vi "CohortRegister.vi"(10 "Action":enum16{"Set", "Get", "Del"}(ring), 11 "Cohort Index":u8) -> (3 "New Index":u8)   [LabVIEW 2012, in "StimulCtrls.lvlib"]
uses:
  StimulCtrls.lvlib
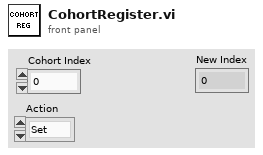
[diagram p1: front panel]
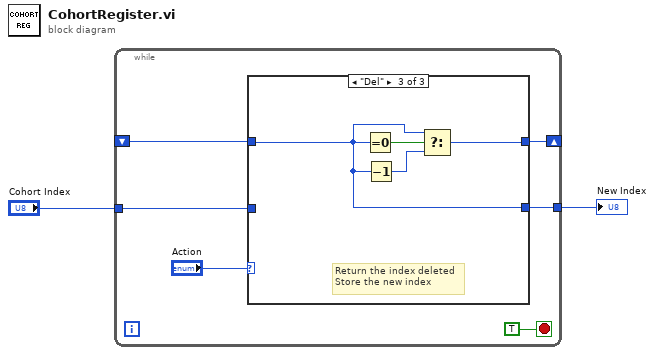
[diagram p0: block diagram]
diagram:
  n1 = while {
    tunnel: "Cohort Index" -> [w4]
    shift-right: [w7] -> _
    shift-left: _ -> [w6]
    tunnel: [w3] -> w1
    stop <- TRUE stop-if-true
    n2 = case shown="\"Del\"" "Action" {
      tunnel: [w9 w10 w12] -> w7
      tunnel: w4 -> [w9 _ _]
      tunnel: w6 -> [_ w10 w11]
      tunnel: [w9 w10 w11] -> w3
      frame "Set", Default {
      }
      frame "Get" {
      }
      frame "Del" {
        # "Return the index deleted\nStore the new index"
        n3 = Equal To 0?(x=w11) -> (x = 0?=w14:bool)
        n4 = Decrement(x=w11) -> (x-1=w13:u8)
        n5 = Select(t=w11, s=w14, f=w13) -> (s? t:f=w12:u8)
      }
    }
  }
  "New Index" <- w1
